vi "Execute.vi"(8 "error in (no error)":errorcluster, 10 "Abstract Consumer in":refnum<class "Abstract Consumer.lvclass">, 11 "Test Message in":refnum<class "Test Message.lvclass">) -> (0 "error out":errorcluster, 1 "Abstract Response out":refnum<class "Abstract Response Message.lvclass">, 2 "Abstract Consumer out":refnum<class "Abstract Consumer.lvclass">, 3 "Test Message out":refnum<class "Test Message.lvclass">, 4 "Stop?":bool)   [LabVIEW 2017, in "Test Message.lvclass"]
uses:
  Test Message.lvclass
  Consumer/Abstract Consumer/Abstract Consumer.lvclass
  Message/Abstract Response Message/Abstract Response Message.lvclass
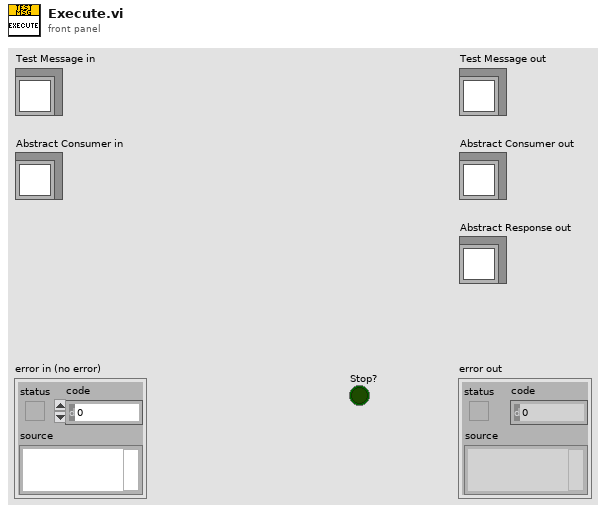
[diagram p1: front panel]
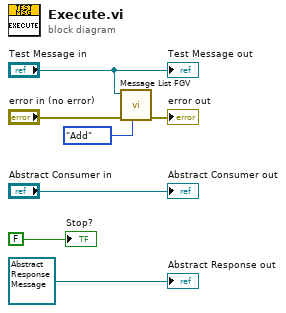
[diagram p0: block diagram]
diagram:
  n1 = call "Message List FGV.vi"("Action (Get)"=enum16{"Get", "Add", "Reset"}."Add", "error in (no error)"="error in (no error)", "Message Object"="Test Message in") -> ("error out"=→"error out":errorcluster)  [unwired: 7 in, 1 out]
  "Test Message out" <- "Test Message in"
  "Abstract Consumer out" <- "Abstract Consumer in"
  "Stop?" <- FALSE ("Stop?")
  "Abstract Response out" <- refnum<class "Abstract Response Message.lvclass"> refnum ("Abstract Response out")
